vi "modbusTxFIFOUpdateLoop.vi"(11 "Modbus Port Settings":T1) -> ()   [LabVIEW 2015]
uses:
  DataTypes/ModbusPortSettings.ctl
  <vilib>/Platform/TimedLoop/XDataNode/timing_clust.ctl
  <vilib>/Platform/TimedLoop/XDataNode/nitl_modes.ctl
  <vilib>/Platform/TimedLoop/XDataNode/wakeup.ctl
  DataTypes/TxInstruction.ctl
  DataTypes/TxInstructionTypes.ctl
  Telemetry/DataTypes/TelemetryUpdateMode.ctl
  <vilib>/rvi/Emulation/niFpgaSctlEmulationGetInTimedLoop.vi
  <vilib>/rvi/Emulation/niFpgaEmulationReportErrorSimple.vi
  <vilib>/rvi/Emulation/niFpgaGetClockAttributes.vi
  <vilib>/rvi/Emulation/niFpgaCriticalErrorInLSC.vi
  <vilib>/rvi/Emulation/niFpgaEmulationIsFPGAContextNoSignature.vi
  <vilib>/rvi/DataTransferAndStorage/Container/Common/niFpgaContainerGetUniqueNameForEmu.vi
  <vilib>/rvi/Memory/Memory_Emulation/niFpgaMemoryEmulationCacheClearOnFirstRun.vi
  <vilib>/rvi/Memory/Memory_Emulation/nirvimemoryEmulationManagerCache_MakeExclusive.vi
  <vilib>/rvi/Memory/Memory_Emulation/niFpgaMemoryEmulationValidateCache.vi
  <vilib>/rvi/Memory/Memory_Emulation/nirvimemoryEmulationManagerCache_InsertValue.vi
  <vilib>/Utility/error.llb/Clear Errors.vi
  <vilib>/rvi/Memory/Memory_Emulation/nirvimemoryEmulationManagerCache_ReleaseExclusive.vi
  <vilib>/rvi/Memory/Memory_Emulation/nirvimemoryEmulationManagerCache_GetValue.vi
  <vilib>/rvi/Memory/Memory_Emulation/nirvimemoryEmulationManagerCache_SetValue.vi
  <vilib>/rvi/Emulation/niFpgaProcessEmulError.vi
  <vilib>/rvi/DataTransferAndStorage/Container/Common/niFpgaContainerExecOnDevCompGetState.vi
  <vilib>/rvi/errors/niFpgaSetErrorForExecOnDevCompSimple.vi
  <vilib>/rvi/eio/common/nirviEmuReportErrorAndStop.vi
  <vilib>/rvi/FIFO/Fifo_Resource/nirvififoEmulationSetSize.vi
  <vilib>/rvi/FIFO/Fifo_Resource/nirviFifoEmulationQueueMgr.vi
  <instcachedir>/0/nirviFifoEmulationQueueMgr_E5CAEC123FF24DC58D834DCA3CDAA9B5.lvgen/nirviFifoEmulationQueueMgr_E5CAEC123FF24DC58D834DCA3CDAA9B5_005.vi
  <vilib>/rvi/FIFO/Fifo_Resource/nirvififoEmulationDetermineInputValidOut.vi
  <vilib>/rvi/FIFO/Fifo_Resource/nirvififoEmulationCreateLock.vi
  <vilib>/rvi/FIFO/Fifo_Resource/nirvififoEmulationObtainLock.vi
  <vilib>/rvi/FIFO/Fifo_Resource/nirvififoEmulationReleaseLock.vi
  <vilib>/rvi/occurrence/nirviWaitOnOccurrenceBase.vi
  <vilib>/rvi/errors/nirviReportUnexpectedCaseInternalError.vi
  <vilib>/rvi/errors/nirviReportUnexpectedCaseInternalError (U32).vi
  <vilib>/rvi/interface/RandomDataEmulation/niFpgaRandomDataHandleErrors.vi
  <instcachedir>/0/nirviFifoEmulationQueueMgr_E5CAEC123FF24DC58D834DCA3CDAA9B5.lvgen/nirviFifoEmulationQueueMgr_E5CAEC123FF24DC58D834DCA3CDAA9B5_010.vi
  <vilib>/Platform/TimedLoop/XDataNode/XDataNode.xnode
  <vilib>/rvi/DataTransferAndStorage/Container/XNode/niFpgaContainer.xnode
  <vilib>/rvi/DataTransferAndStorage/Register/Emulation/niFpgaRegisterEmulation.vi
  <vilib>/rvi/FIFO/Fifo_Resource/niFpgaFifoEmulationRefIn.vi
  <vilib>/Platform/TimedLoop/XDataNode/XDNodeRunTimeDep.lvlib
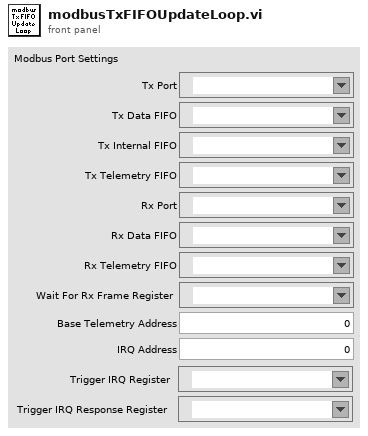
[diagram p1: front panel]
types:
  T1 = typedef "ModbusPortSettings.ctl" = cluster{"Tx Port":refnum<k21>, "Tx Data FIFO":refnum<k21>, "Tx Internal FIFO":refnum<k21>, "Tx Telemetry FIFO":refnum<k21>, "Rx Port":refnum<k21>, "Rx Data FIFO":refnum<k21>, "Rx Telemetry FIFO":refnum<k21>, "Base Telemetry Address":u32, "Wait For Rx Frame Register":refnum<k21>, "IRQ Address":u8, "Trigger IRQ Register":refnum<k21>, "Trigger IRQ Response Register":refnum<k21>}
  T2 = typedef "XDNodeRunTimeDep.lvlib/timing_clust.ctl" = cluster{"Expected End [f-1]":u64, "Actual End [f-1]":u64, "Finished Late? [f-1]":bool, "Expected End [i-1]":u64, "Actual End [i-1]":u64, "Finished Late? [i-1]":bool, "Expected Start [i]":u64, "Actual Start [i]":u64, "Expected Start [f]":u64, "Actual Start [f]":u64, "Source Name":string, "Structure Name":string, "Period":i64, "Deadline":i64, "Offset":i64, "Start":i64, "Priority":i32, "Timeout":i32, "Mode":T3, "Wakeup Reason":T4, "Error":errorcluster, "Source Type":string, "Secondary Source Type":string, "Global End Time":u64, "Global Start Time":u64, "Frame Duration":u64, "Iteration Duration":u64, "Assigned CPU":i32, "I/O Scan Engine Mode":u32}
  T3 = typedef "XDNodeRunTimeDep.lvlib/nitl_modes.ctl" = enum32{"No Change", "Process missed periods, maintain original phase", "Discard missed periods, maintain original phase", "Process missed periods, ignore original phase", "Discard missed periods, ignore original phase"}
  T4 = typedef "XDNodeRunTimeDep.lvlib/wakeup.ctl" = enum32{"Normal", "Aborted", "Asynchronous wakeup", "Timing source error", "Timed loop error", "Timeout"}
  T5 = typedef "TxInstruction.ctl" = cluster{"Tx Instruction Type":T6, "Data":u16}
  T6 = typedef "TxInstructionTypes.ctl" = enum8{"NOP", "WriteByte", "EndOfFrame", "DelayTicks", "DelayMicroseconds", "DelayMilliseconds", "WaitForRxFrame", "TriggerIRQ"}
  T7 = typedef "TelemetryUpdateMode.ctl" = enum8{"NOP", "Set", "Add", "Subtract", "Or"}
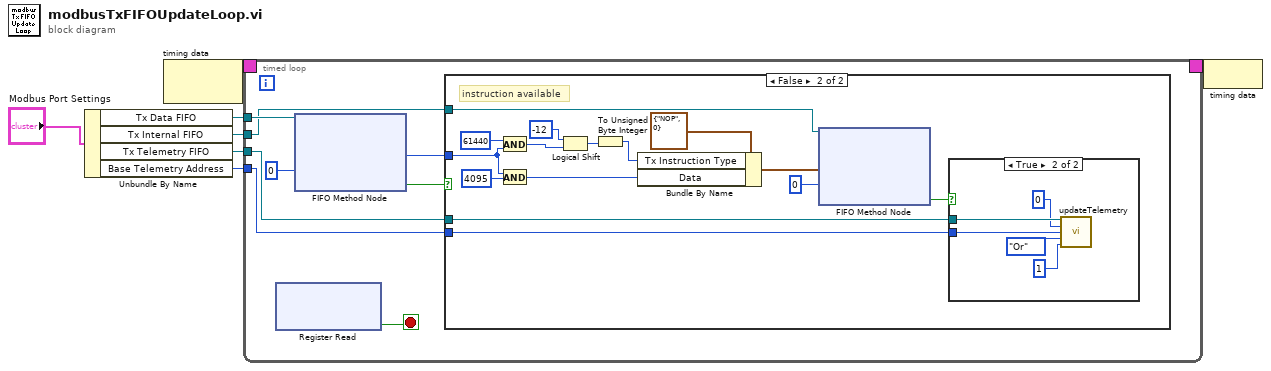
[diagram p0: block diagram]
diagram:
  n1 = Unbundle By Name("Modbus Port Settings") -> ("Tx Data FIFO"=w4:refnum<k21>, "Tx Internal FIFO"=w5:refnum<k21>, "Tx Telemetry FIFO"=w2:refnum<k21>, "Base Telemetry Address"=w1:u32)
  n2 = node-c288() -> (w7:T2)  [unwired: 1 in]
  n3 = timed-loop {
    timing: w7 -> [_]
    timing-out: [_] -> w6
    tunnel: w4 -> [w15]
    tunnel: w5 -> [w11]
    tunnel: w2 -> [w9]
    tunnel: w1 -> [w8]
    stop <- w10 stop-if-true
    n4 = xnode ("Register Read")() -> ("Data"=w10:bool)  [unwired: 1 in, 1 out]
    n5 = xnode ("FIFO Method Node")("Timeout"=0, "FIFO In"=w15) -> ("Element"=w12:u16, "Timed Out?"=w13:bool)  [unwired: 1 out]
    n6 = case shown="False" w13 {
      tunnel: w12 -> [_ w20]
      tunnel: w11 -> [_ w23]
      tunnel: w9 -> [_ w17]
      tunnel: w8 -> [_ w16]
      frame True {
        # "no instruction available"
      }
      frame False {
        # "instruction available"
        n7 = And(x=u16 61440 ("y"), y=w20) -> (x .and. y?=w29:u16)
        n8 = And(x=w20, y=u16 4095) -> (x .and. y?=w25:u16)
        n9 = Logical Shift(y=i16 -12, x=w29) -> (x << y=w27:u16)
        n10 = To Unsigned Byte Integer(number=w27) -> (unsigned 8bit integer=w24:u8)
        n11 = Bundle By Name(cluster=T5 {"Tx Instruction Type"=enum."NOP", "Data"=0} ("Tx Instruction"), "Tx Instruction Type"=w24, "Data"=w25) -> (w22:T5)
        n12 = xnode ("FIFO Method Node")("Element"=w22, "Timeout"=0, "FIFO In"=w23) -> ("Timed Out?"=w18:bool)  [unwired: 1 out]
        n13 = case shown="True" w18 {
          tunnel: w17 -> [_ w35]
          tunnel: w16 -> [_ w34]
          frame False {
          }
          frame True {
            n14 = call "updateTelemetry.vi"("Telemetry FIFO"=w35, "Address Offset"=u32 0, "Base Address"=w34, "Telemetry Update Mode"=TelemetryUpdateMode."Or", "Data"=u32 1) -> ()  [unwired: 11 in]
          }
        }
      }
    }
  }
  n15 = node-c288(w6) -> ()
